vi "Get reference[].vi"(8 "error in (no error)":errorcluster, 11 "LV MDI in":refnum<class "LV MDI.lvclass">) -> (0 "error out":errorcluster, 2 "Reference[]":refnum<vi>[](array[refnum]), 3 "LV MDI out":refnum<class "LV MDI.lvclass">)   [LabVIEW 2016, in "LV MDI.lvclass"]
doc: "Get all child window reference."
uses:
  LV MDI.lvclass
  LV MDI.lvclass/LV MDI.ctl
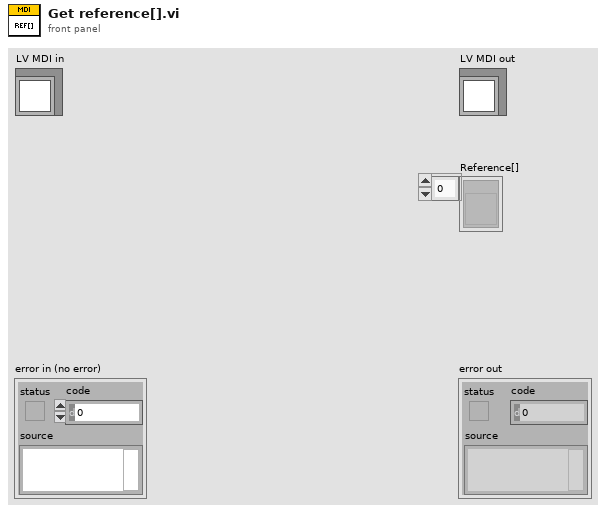
[diagram p1: front panel]
types:
  T1 = typedef "LV MDI.lvclass/Child Window Data.ctl" = cluster{"Child hWnd":u32, "UID":string, "vi reference":refnum<vi>, "Name":string}
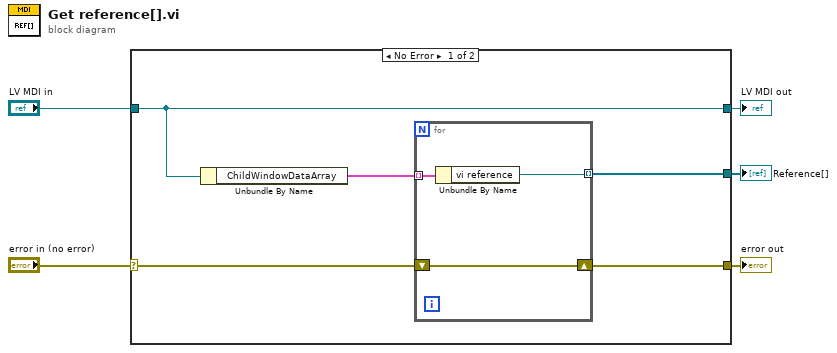
[diagram p0: block diagram]
diagram:
  n1 = case shown="No Error" "error in (no error)" {
    selector: "error in (no error)" -> [w9 w15]
    tunnel: [w8 w15] -> w4
    tunnel: [w10 w14] -> w2
    tunnel: "LV MDI in" -> [w10 w14]
    tunnel: [w6 _] -> w1
    frame No Error {
      n2 = Unbundle By Name(w10) -> ("ChildWindowDataArray"=w7:T1[])
      n3 = for {
        shift-right: [w13] -> w8
        shift-left: w9 -> [w13]
        tunnel: w7 -> [w12] mode=indexing
        tunnel: [w11] -> w6 mode=indexing
        n4 = Unbundle By Name(w12) -> ("vi reference"=w11:refnum<vi>)
      }
    }
    frame Error {
    }
  }
  "error out" <- w4
  "LV MDI out" <- w2
  "Reference[]" <- w1
